vi "Dashboard Main.vi"() -> ()   [LabVIEW 2013]
uses:
  robot/util/telemetry.ctl
  robot/util/inputs.ctl
  robot/drive/drive_inputs.ctl
  robot/flinger/flinger_inputs.ctl
  robot/roller/roller_inputs.ctl
  robot/util/outputs.ctl
  robot/drive/drive_outputs.ctl
  robot/flinger/flinger_outputs.ctl
  <vilib>/Rock Robotics/WPI/Solenoid/WPI_SolenoidValue.ctl
  robot/roller/roller_outputs.ctl
panel:
  out "Roller Output":dbl(slide) scale=-12.0..12.0
  out "Sol_Position":T1
  out "Solenoid Value":T1
  out "Roller Set Speed":dbl(slide) scale=-12.0..12.0
  in  "Telemetry":T2
  out "Battery":sgl
  out "Robot IP Address":string="10.0.0.2"
  out "Status":T11(ring)
  out "Snake!":cluster{"X":dbl, "Y":dbl}[](graph) caption="Remember to robot occasionally!"
  in  "Hide the\nsnakes?":bool
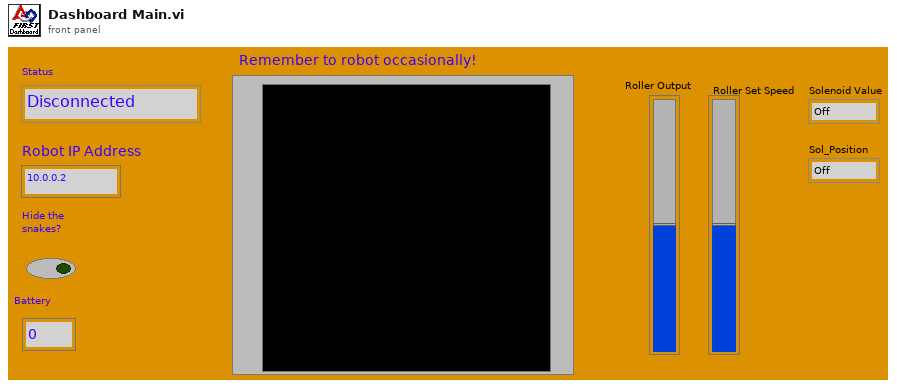
[diagram p1: front panel]
types:
  T1 = typedef "WPI_SolenoidValue.ctl" = enum16{"Off", "On", "Forward", "Reverse"}
  T2 = typedef "telemetry.ctl" = cluster{"Inputs":T3, "Outputs":T7}
  T3 = typedef "inputs.ctl" = cluster{"Drive_inputs":T4, "Flinger Inputs":T5, "Roller Inputs":T6}
  T4 = typedef "drive_inputs.ctl" = cluster{"j_x":dbl, "j_y":dbl, "Heading":dbl}
  T5 = typedef "flinger_inputs.ctl" = cluster{"Shoot":bool, "Power":dbl, "Override":bool}
  T6 = typedef "roller_inputs.ctl" = cluster{"Arm_In":bool, "Motor_On":bool, "Motor_Velocity":dbl}
  T7 = typedef "outputs.ctl" = cluster{"Drive_Outputs":T8, "Flinger Outputs":T9, "Roller_Outputs":T10}
  T8 = typedef "drive_outputs.ctl" = cluster{"left":dbl, "right":dbl}
  T9 = typedef "flinger_outputs.ctl" = cluster{"Solenoid Value":T1}
  T10 = typedef "roller_outputs.ctl" = cluster{"Sol_Position":T1, "Motor_Voltage":dbl}
  T11 = enum8{"Disconnected", "E-Stop", "Disabled", "Enabled"}
  T12 = cluster{"Competition mode":bool, "Robot Link":bool, "Autonomous":bool, "Enabled":bool, "E-Stop":bool}
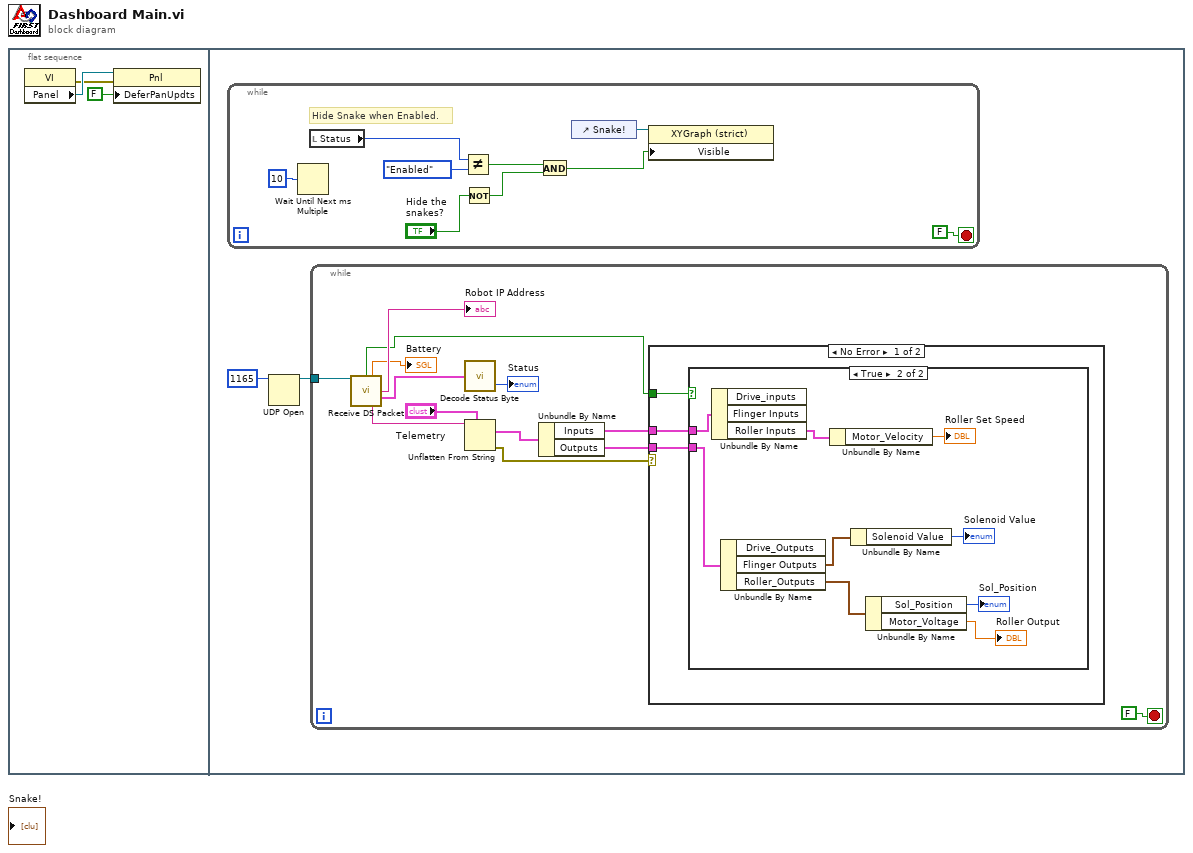
[diagram p0: block diagram]
diagram:
  n1 = flat-sequence {
    frame #0 {
      n2 = property class="VI"() -> (error out=w2:errorcluster, "Panel"=w3:refnum<vi>)  [unwired: 2 in, 1 out]
      n3 = property class="Pnl"(reference=w3, error in=w2, "DeferPanUpdts"=FALSE) -> ()  [unwired: 2 out]
    }
    frame #1 {
      n4 = while {
        stop <- FALSE stop-if-true
        # "Hide Snake when Enabled."
        n5 = Wait Until Next ms Multiple(millisecond multiple=u32 10) -> ()  [unwired: 1 out]
        n6 = local read "Status"() -> (w31:T11)
        n7 = Not Equal?(x=w31, y=T11."Enabled" ("Status")) -> (x != y?=w38:bool)
        n8 = Not(x="Hide the\nsnakes?") -> (.not. x?=w37:bool)
        n9 = And(x=w38, y=w37) -> (x .and. y?=w36:bool)
        n10 = control-ref of="Snake!"() -> (w32:refnum<vi>)
        n11 = property class="XYGraph (strict)"(reference=w32, "Visible"=w36) -> ()  [unwired: 1 in, 2 out]
      }
      n12 = UDP Open(11:u16 1165 ("port")) -> (port=w4:refnum<k16>)  [unwired: 2 in, 4 out]
      n13 = while {
        tunnel: w4 -> [w17]
        stop <- FALSE stop-if-true
        n14 = call "Receive DS Packet.vi"("Recv Socket"=w17) -> ("New Dashboard Data"=w9:bool, "Battery"=→"Battery":sgl, "Robot IP Address"=→"Robot IP Address":string, "Status"=w16:T12, "High Priority User Data"=w12:string)  [unwired: 1 in, 9 out]
        n15 = call "Decode Status Byte.vi"("Status Byte"=w16) -> ("Status"=→"Status":T11)  [unwired: 1 out]
        n16 = Unflatten From String(type="Telemetry", binary string=w12) -> (value=w11:T2, error out=w10:errorcluster)  [unwired: 3 in, 1 out]
        n17 = Unbundle By Name(w11) -> ("Inputs"=w8:T3, "Outputs"=w7:T7)
        n18 = case shown="No Error" w10 {
          tunnel: w9 -> [w21 _]
          tunnel: w8 -> [w20 _]
          tunnel: w7 -> [w19 _]
          frame No Error {
            n19 = case shown="True" w21 {
              tunnel: w20 -> [_ w27]
              tunnel: w19 -> [_ w30]
              frame False {
              }
              frame True {
                n20 = Unbundle By Name(w27) -> ("Roller Inputs"=w26:T6)  [unwired: 2 out]
                n21 = Unbundle By Name(w30) -> ("Flinger Outputs"=w29:T9, "Roller_Outputs"=w28:T10)  [unwired: 1 out]
                n22 = Unbundle By Name(w26) -> ("Motor_Velocity"=→"Roller Set Speed":dbl)
                n23 = Unbundle By Name(w29) -> ("Solenoid Value"=→"Solenoid Value":T1)
                n24 = Unbundle By Name(w28) -> ("Sol_Position"=→"Sol_Position":T1, "Motor_Voltage"=→"Roller Output":dbl)
              }
            }
          }
          frame Error {
          }
        }
      }
    }
  }
